vi "fgv_9221-config.vi"(7 "cmd":T2, 8 "error in":errorcluster, 11 "cDAQ 9221 Config":T1={"input terminal"=10083, "minimum value"=-60.0, "maximum value"=60.0, "number of samples"=1000, "rate"=10000.0, "sample mode"=10123, "physical channels"=""} {"sample mode" items=["Finite Samples"=10178, "Continuous Samples"=10123, "Hardware Timed Single Point"=12522]; "rate" format="%0.2f"; "maximum value" format="%^.2e"; "minimum value" format="%^.2e"; "input terminal" items=["default"=-1, "RSE"=10083, "NRSE"=10078, "Differential"=10106, "Pseudodifferential"=12529]}) -> (0 "error out":errorcluster, 3 "cDAQ 9221 Config 2":T1={"input terminal"=10083, "minimum value"=-60.0, "maximum value"=60.0, "number of samples"=1000, "rate"=10000.0, "sample mode"=10123, "physical channels"=""} {"sample mode" items=["Finite Samples"=10178, "Continuous Samples"=10123, "Hardware Timed Single Point"=12522]; "rate" format="%0.2f"; "maximum value" format="%^.2e"; "minimum value" format="%^.2e"; "input terminal" items=["default"=-1, "RSE"=10083, "NRSE"=10078, "Differential"=10106, "Pseudodifferential"=12529]})   [LabVIEW 2019]
uses:
  _ctrl/rw.ctl
  Set_NIAI.ctl
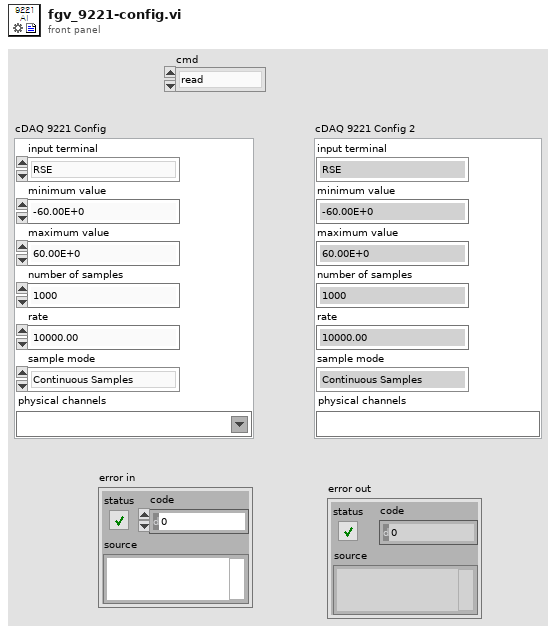
[diagram p1: front panel]
types:
  T1 = typedef "Set_NIAI.ctl" = cluster{"input terminal":i32, "minimum value":dbl, "maximum value":dbl, "number of samples":i32, "rate":dbl, "sample mode":i32, "physical channels":tag}
  T2 = typedef "rw.ctl" = enum16{"read", "write"}
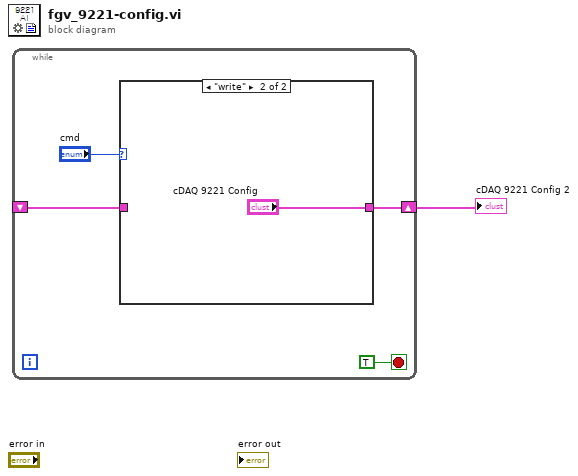
[diagram p0: block diagram]
diagram:
  n1 = while {
    shift-right: [w3] -> w1
    shift-left: _ -> [w2]
    stop <- TRUE stop-if-true
    n2 = case shown="\"write\"" "cmd" {
      tunnel: [w6 "cDAQ 9221 Config"] -> w3
      tunnel: w2 -> [w6 _]
      frame "read", Default {
      }
      frame "write" {
      }
    }
  }
  "cDAQ 9221 Config 2" <- w1
